vi "WPI_CameraSend Images to PC Loop_ONELOOP.vi"(6 "CameraDevRef Back":T1, 8 "error in (no error)":errorcluster, 9 "port":u16, 10 "Image Name":string, 11 "CameraDevRef Front":T1) -> ()   [LabVIEW 2015]
doc: "This VI is used to send images to the dashboard using the second enet port on the 8 slot controller. This is provided for compatibility, but is higher overhead than using the Camera MJPG approach.\n\nThis software is licensed. Open the labview\\readme\\WPI Robotics Library Open Source License.txt file for more information."
uses:
  <vilib>/Rock Robotics/WPI/Camera/WPI_CameraDevRef.ctl
  <vilib>/Rock Robotics/SystemInterfaces/NetworkCommunication/NetComm_UsageReport_ResourceType.ctl
  <vilib>/Rock Robotics/Network Tables/NT Read Boolean.vi
  Global Variables/Temp Variables.vi
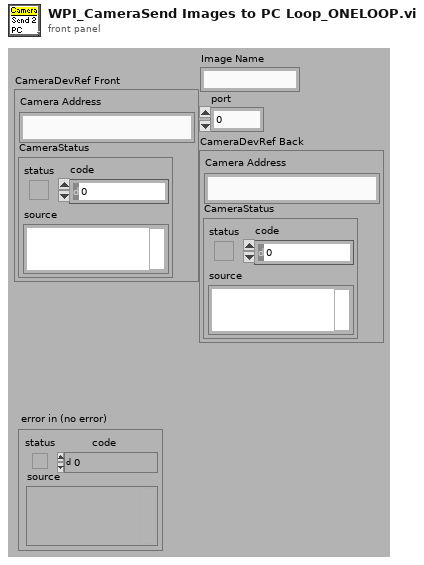
[diagram p1: front panel]
types:
  T1 = typedef "WPI_CameraDevRef.ctl" = cluster{"Camera Address":string, "CameraStatus":errorcluster}
  T2 = cluster{"fps":i32, "compression":i32, "compression 2":i32}
  T3 = typedef "NetComm_UsageReport_ResourceType.ctl" = enum8{"Controller", "Module", "Language", "CANPlugin", "Accelerometer", "ADXL345", "AnalogChannel", "AnalogTrigger", "AnalogTriggerOutput", "CANJaguar", "Compressor", "Counter", "Dashboard", "DigitalInput", "DigitalOutput", "DriverStationCIO", "DriverStationEIO", "DriverStationLCD", "Encoder", "GearTooth", "Gyro", "I2C", "Framework", "Jaguar", "Joystick", "Kinect", "KinectStick", "PIDController", "Preferences", "PWM", "Relay", "RobotDrive", "SerialPort", "Servo", "Solenoid", "SPI", "Task", "Ultrasonic", "Victor", "Button", "Command", "AxisCamera", "PCVideoServer", "SmartDashboard", "Talon", "HiTechnicColorSensor", "HiTechnicAccel", "HiTechnicCompass", "SRF08", "AnalogOutput", "Victor SP", "Talon SRX", "CAN Talon SRX", "ADXL362 Accel", "ADXRS450 Gyro", "Rev SPARK", "Mindsensors SD540", "Digital Filter"}
  T4 = enum16{"Update Mode", "Get Image", "Get Image Data"}
  T5 = typedef "Image Type" = u32
  T6 = typedef "IMAQ Image.ctl" = refnum<image>
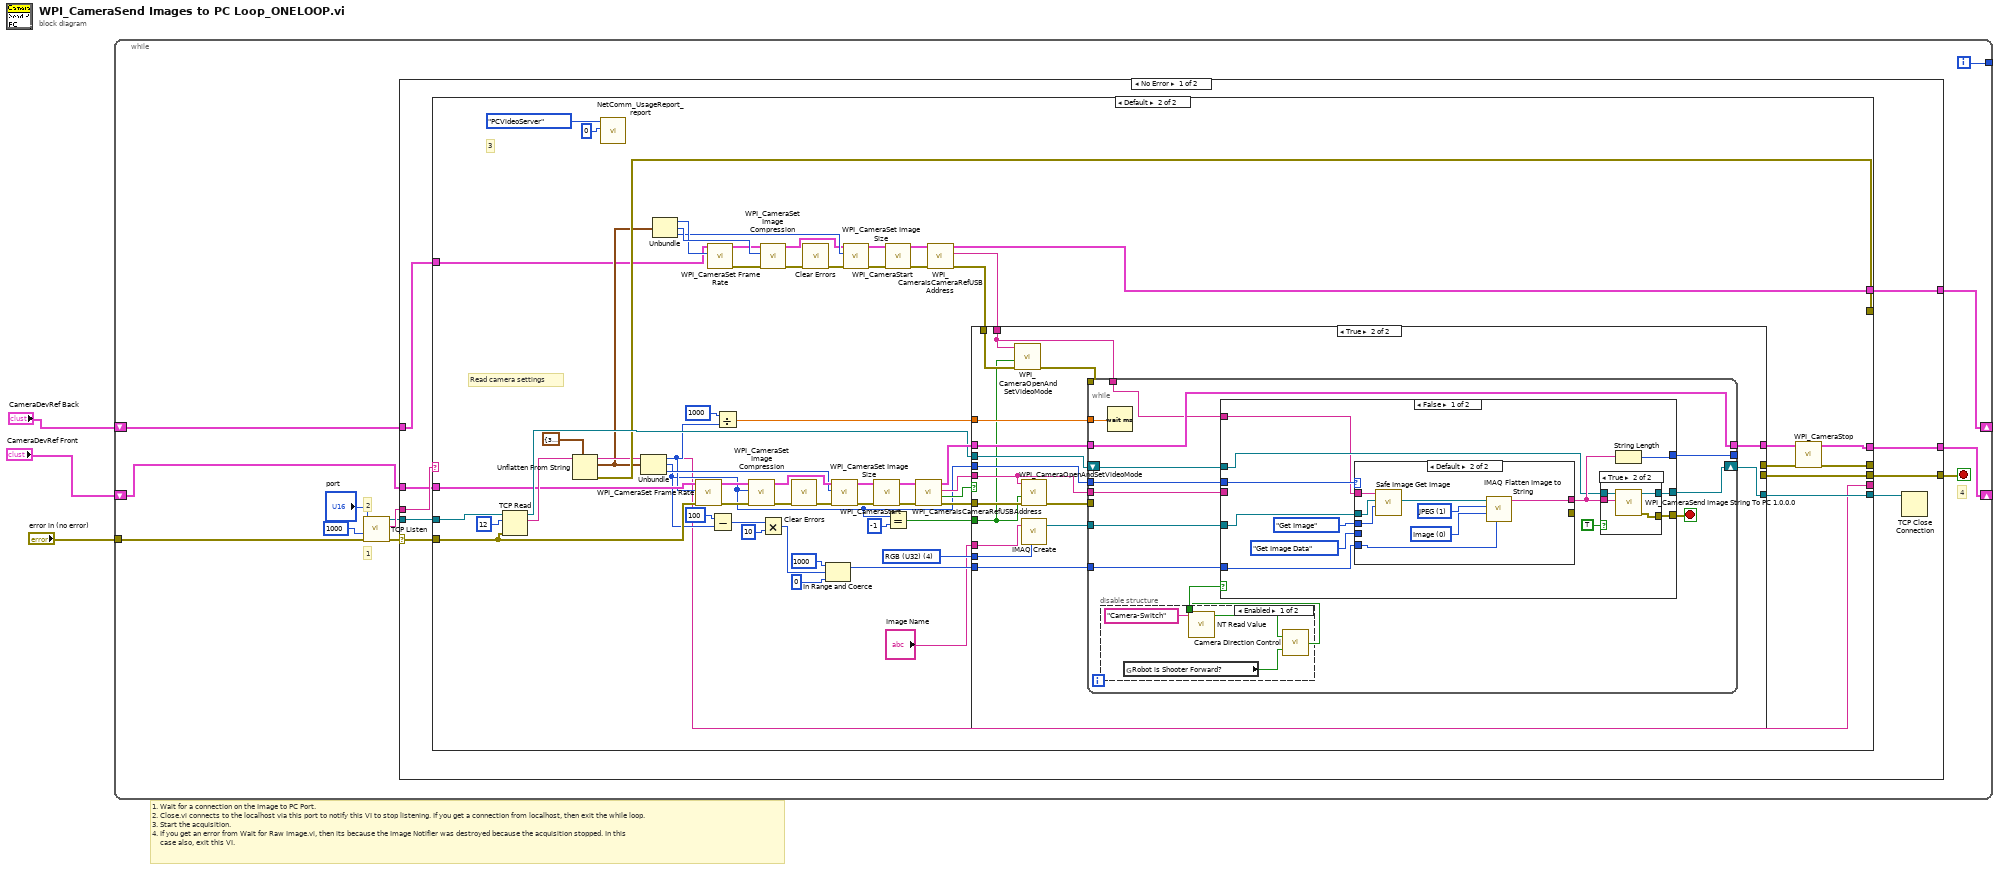
[diagram p0: block diagram]
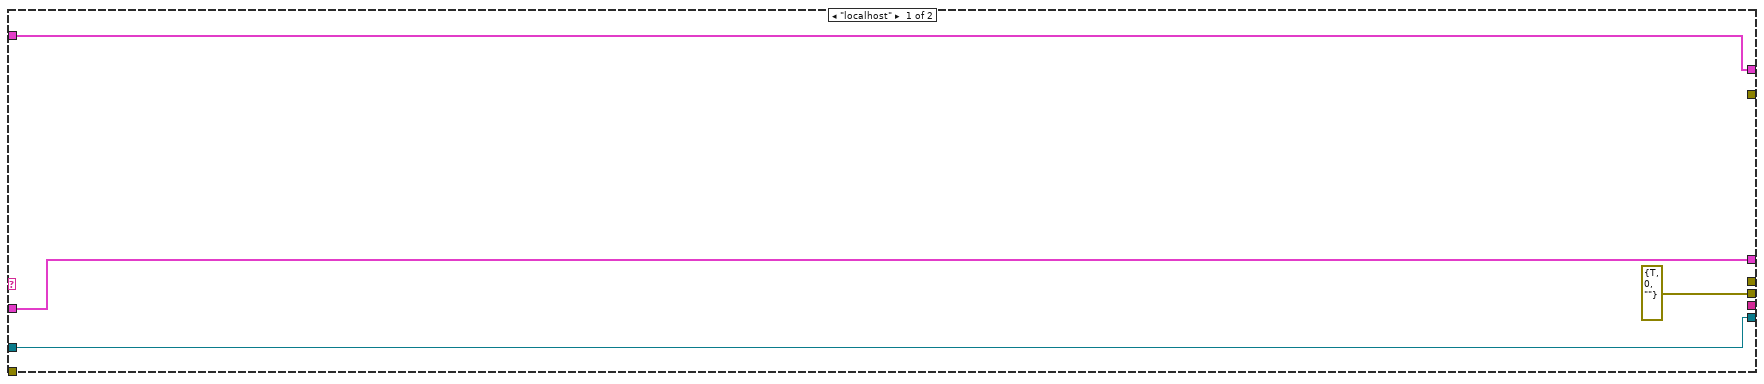
[diagram p2: hidden frame]
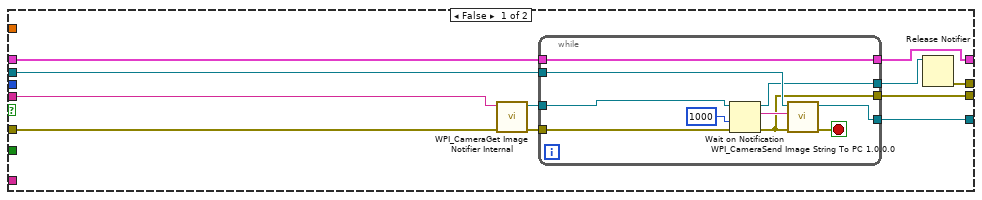
[diagram p3: hidden frame]
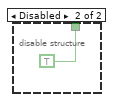
[diagram p4: hidden frame]
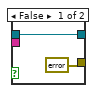
[diagram p5: hidden frame]
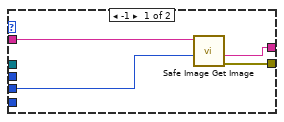
[diagram p6: hidden frame]
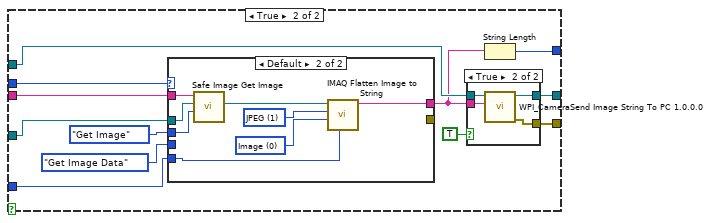
[diagram p7: hidden frame]
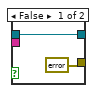
[diagram p8: hidden frame]
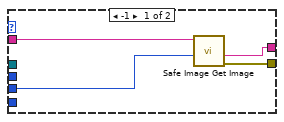
[diagram p9: hidden frame]
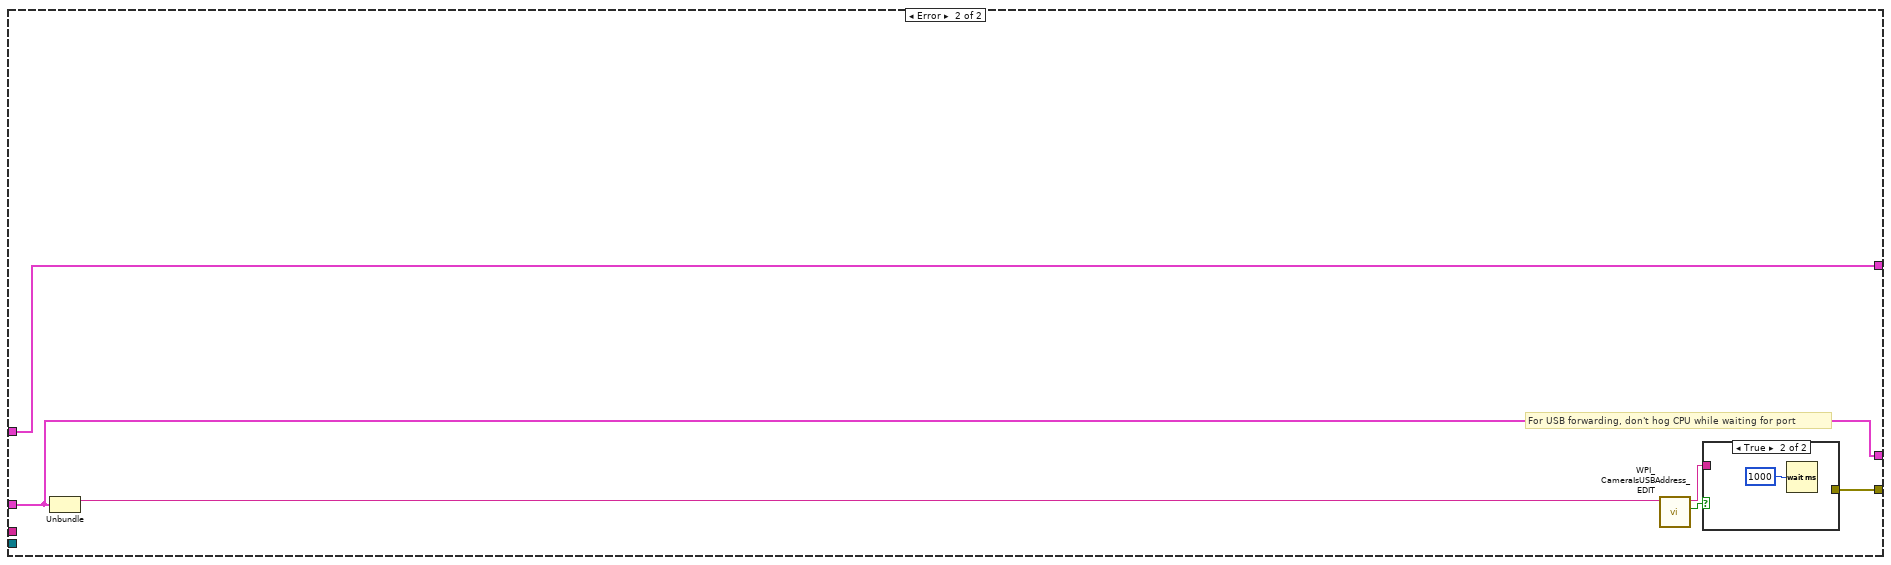
[diagram p10: hidden frame]
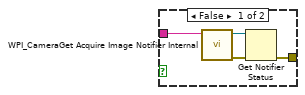
[diagram p11: hidden frame]
diagram:
  # "1. Wait for a connection on the Image to PC Port.\n2. Close.vi connects to the localhost via this port to notify this VI to stop listening. If you get a connection from localhost, then exit the while loop.\n3. Start the acquisition.\n4. If you get an error from Wait for Raw Image.vi, then its because the Image Notifier was destroyed because the acquisition stopped. In this\n    case also, exit this VI."
  n1 = while {
    tunnel: "error in (no error)" -> [w13]
    shift-right: [w15] -> _
    shift-left: "CameraDevRef Front" -> [w7]
    tunnel: [w8] -> _
    shift-right: [w4] -> _
    shift-left: "CameraDevRef Back" -> [w5]
    i -> [w8]
    stop <- w11 stop-if-true
    # "4"
    # "1"
    # "2"
    n2 = call <vilib>:"TCP Listen.vi"("error in (no error)"=w13, "timeout ms (wait forever: -1)"=u16 1000 ("port"), "port"="port") -> ("error out"=w10:errorcluster, "remote address"=w14:string, "connection ID"=w12:refnum<k5>)  [unwired: 1 in, 5 out]
    n3 = case shown="No Error" w10 {
      selector: w10 -> [w18 _]
      tunnel: [w24 w211] -> w15
      tunnel: w14 -> [w23 _]
      tunnel: w7 -> [w22 w211]
      tunnel: w12 -> [w21 _]
      tunnel: [w20 w212] -> w11
      tunnel: w5 -> [w17 w207]
      tunnel: [w16 w207] -> w4
      frame No Error {
        n4 = case shown="Default" w23 {
          tunnel: [w28 w89] -> w24
          tunnel: w22 -> [w28 w72]
          tunnel: w18 -> [_ w68]
          tunnel: w21 -> [w26 w76]
          tunnel: [errorcluster {"status"=TRUE, "code"=0, "source"=""} ("error out 2") w91] -> w20
          tunnel: [w26 w90] -> w19
          tunnel: [_ w88] -> _
          tunnel: [_ w48] -> _
          tunnel: [_ w47] -> _
          tunnel: w17 -> [w25 w32]
          tunnel: [w25 w29] -> w16
          frame "localhost" {
          }
          frame Default {
            w83 = T5 4 items=["Grayscale (U8)", "Grayscale (I16)", "Grayscale (SGL)", "Complex (CSG)", "RGB (U32)", "HSL (U32)", "RGB (U64)", "Grayscale (U16)"] ("Image Type")
            # "Read camera settings"
            # "3"
            n5 = TCP Read(connection ID=w76, bytes to read=12, error in (no error)=w68) -> (connection ID out=w75:refnum<k5>, data out=w73:string)  [unwired: 2 in, 1 out]
            n6 = Unflatten From String(type=T2 {"fps"=30, "compression"=32, "compression 2"=32} ("Camera Settings"), binary string=w73) -> (rest of the binary string=w47:string, value=w33:T2, error out=w48:errorcluster)  [unwired: 3 in]
            n7 = call <vilib>:"NetComm_UsageReport_report.vi"("Instance Number"=u8 0, "Resource Type"=NetComm_UsageReport_ResourceType."PCVideoServer") -> ()  [unwired: 10 in]
            n8 = Unbundle(w33) -> ("fps"=w63:i32, "compression"=w52:i32, "compression 2"=w65:i32)
            n9 = Unbundle(w33) -> ("fps"=w42:i32, "compression"=w43:i32, "compression 2"=w41:i32)
            n10 = call <vilib>:"WPI_CameraSet Frame Rate.vi"("error in (no error)"=w68, "Frame Rate (fps)"=w63, "CameraDevRef"=w72) -> ("error out"=w67:errorcluster, "CameraDevRef Out"=w71:T1)  [unwired: 7 in]
            n11 = call <vilib>:"WPI_CameraSet Frame Rate.vi"("Frame Rate (fps)"=w42, "CameraDevRef"=w32) -> ("error out"=w39:errorcluster, "CameraDevRef Out"=w36:T1)  [unwired: 8 in]
            n12 = Subtract(x=100, y=w52) -> (x-y=w57:i32)
            n13 = Divide(x=u16 1000 ("port"), y=w63) -> (x/y=w62:dbl)
            n14 = call <vilib>:"WPI_CameraSet Image Compression.vi"("error in (no error)"=w67, "Compression"=w52, "CameraDevRef"=w71) -> ("error out"=w50:errorcluster, "CameraDevRef Out"=w70:T1)  [unwired: 7 in]
            n15 = call <vilib>:"WPI_CameraSet Image Compression.vi"("error in (no error)"=w39, "Compression"=w43, "CameraDevRef"=w36) -> ("error out"=w44:errorcluster, "CameraDevRef Out"=w37:T1)  [unwired: 7 in]
            n16 = Multiply(x=w57, y=10) -> (x*y=w59:i32)
            n17 = call <vilib>:"Clear Errors.vi"("error in (no error)"=w50) -> ("error out"=w49:errorcluster)  [unwired: 5 in, 1 out]
            n18 = call <vilib>:"Clear Errors.vi"("error in (no error)"=w44) -> ("error out"=w45:errorcluster)  [unwired: 5 in, 1 out]
            n19 = In Range and Coerce(upper limit=1000, x=w59, lower limit=0) -> (coerced(x)=w55:i32)  [unwired: 1 out]
            n20 = call <vilib>:"WPI_CameraSet Image Size.vi"("error in (no error)"=w49, "Image Size"=w65, "CameraDevRef"=w70) -> ("error out"=w66:errorcluster, "CameraDevRef Out"=w69:T1)  [unwired: 7 in]
            n21 = call <vilib>:"WPI_CameraSet Image Size.vi"("error in (no error)"=w45, "Image Size"=w41, "CameraDevRef"=w37) -> ("error out"=w40:errorcluster, "CameraDevRef Out"=w38:T1)  [unwired: 7 in]
            n22 = call <vilib>:"WPI_CameraStart.vi"("error in (no error)"=w66, "CameraDevRef"=w69) -> ("error out"=w80:errorcluster, "CameraDevRef"=w78:T1)  [unwired: 8 out]
            n23 = call <vilib>:"WPI_CameraStart.vi"("error in (no error)"=w40, "CameraDevRef"=w38) -> ("error out"=w34:errorcluster, "CameraDevRef"=w35:T1)  [unwired: 8 out]
            n24 = Equal?(x=w52, y=-1) -> (x = y?=w51:bool)
            n25 = call <vilib>:"WPI_CameraIsCameraRefUSBAddress.vi"("error in (no error)"=w80, "CameraDevRef"=w78) -> ("error out"=w79:errorcluster, "USB?"=w81:bool, "Camera Address Out"=w82:string, "CameraDevRef out"=w77:T1)  [unwired: 6 in]
            n26 = call <vilib>:"WPI_CameraIsCameraRefUSBAddress.vi"("error in (no error)"=w34, "CameraDevRef"=w35) -> ("error out"=w30:errorcluster, "Camera Address Out"=w31:string, "CameraDevRef out"=w29:T1)  [unwired: 6 in, 1 out]
            n27 = case shown="True" w81 {
              tunnel: w75 -> [w102 w129]
              tunnel: [w101 _] -> w91
              tunnel: [w100 w128] -> w90
              tunnel: w79 -> [w99 w120]
              tunnel: w82 -> [w97 w119]
              tunnel: [w96 w124] -> w87
              tunnel: w77 -> [w95 w125]
              tunnel: [w93 _] -> w86
              tunnel: w83 -> [_ w126]
              tunnel: w55 -> [_ w123]
              tunnel: w62 -> [_ w122]
              tunnel: w52 -> [_ w121]
              tunnel: w51 -> [_ w115]
              tunnel: "Image Name" -> [_ w117]
              tunnel: w31 -> [_ w113]
              tunnel: w30 -> [_ w116]
              frame False {
                n28 = call <vilib>:"WPI_CameraGet Image Notifier Internal.vi"("error in (no error)"=w99, "Camera Address"=w97) -> ("error out"=w98:errorcluster, "Image Notifier"=w94:refnum<notifier>)  [unwired: 8 out]
                n29 = while {
                  tunnel: w98 -> [w108]
                  tunnel: w102 -> [w112]
                  tunnel: [w105] -> w101
                  tunnel: [w110] -> w100
                  tunnel: [w109] -> w96
                  tunnel: w95 -> [w109]
                  tunnel: w94 -> [w107]
                  tunnel: [w103] -> w92
                  stop <- w111 stop-if-true
                  n30 = Wait on Notification(notifier=w107, timeout in ms (-1)=1000 ("Timeout in ms (-1)"), error in (no error)=w108) -> (notifier out=w103:refnum<notifier>, notification=w106:string, error out=w105:errorcluster)  [unwired: 2 out]
                  n31 = call <vilib>:"WPI_CameraSend Image String To PC 1.0.0.0.vi"("error in (no error)"=w105, "String"=w106, "TCP Connection ID"=w112) -> ("error out"=w111:errorcluster, "TCP Connection ID out"=w110:refnum<k5>)  [unwired: 7 out]
                }
                n32 = Release Notifier(notifier=w92) -> (error out=w93:errorcluster)  [unwired: 1 in, 3 out]
              }
              frame True {
                n33 = call <vilib>:"WPI_CameraOpenAndSetVideoMode.vi"("error in (no error)"=w116, "USB JPEG"=w115, "Camera Address Out"=w113) -> ("error out"=w114:errorcluster)  [unwired: 8 in]
                n34 = call <vilib>:"WPI_CameraOpenAndSetVideoMode.vi"("error in (no error)"=w120, "USB JPEG"=w115, "Camera Address Out"=w119) -> ("error out"=w118:errorcluster)  [unwired: 8 in]
                n35 = call "IMAQ Create"("Image Name"=w117, "Image Type"=w126) -> ("New Image"=w127:T6)  [unwired: 3 in, 1 out]
                n36 = while {
                  tunnel: w119 -> [w140]
                  shift-right: [w141] -> w128
                  shift-left: w129 -> [w136]
                  tunnel: w127 -> [w139]
                  tunnel: [w132] -> w124
                  tunnel: w125 -> [w132]
                  tunnel: w123 -> [w138]
                  tunnel: w122 -> [w137]
                  tunnel: [w135] -> _
                  tunnel: w121 -> [w134]
                  tunnel: w118 -> [_]
                  tunnel: w114 -> [_]
                  tunnel: w113 -> [w131]
                  stop <- w133 stop-if-true
                  n37 = disable-structure shown="Enabled" {
                    disable-tunnel: [w142 TRUE] -> w130
                    frame Enabled {
                      n38 = global read "Temp Variables.vi" "Robot is Shooter Forward?"() -> (w144:bool)
                      n39 = call-poly <vilib>:"NT Read Value.vi"("Name"="Camera-Switch") -> ("Boolean"=w143:bool)  [unwired: 9 in, 1 out]
                      n40 = call "Camera Direction Control.vi"("Current Driving Direction (True = Shooter Forward)"=w144, "Camera Switch"=w143) -> ("Camera Direction (True = Shooter Camera)"=w142:bool)
                    }
                    frame Disabled {
                    }
                  }
                  n41 = Wait (ms)(milliseconds to wait=w137) -> ()  [unwired: 1 out]
                  n42 = case shown="False" w130 {
                    tunnel: [w149 w188] -> w141
                    tunnel: w140 -> [_ w187]
                    tunnel: w139 -> [w153 w186]
                    tunnel: w138 -> [w154 w185]
                    tunnel: w136 -> [w152 w184]
                    tunnel: [w150 w183] -> w135
                    tunnel: w134 -> [w151 w182]
                    tunnel: [w147 w179] -> w133
                    tunnel: w131 -> [w148 _]
                    frame False {
                      n43 = case shown="Default" w151 {
                        tunnel: [w167 w176] -> w157
                        tunnel: w148 -> [w168 w172]
                        tunnel: w153 -> [_ w171]
                        tunnel: w154 -> [_ w173]
                        tunnel: [w166 _] -> _
                        tunnel: T4."Get Image Data" ("Operation") -> [w165 _]
                        tunnel: T4."Get Image" ("Operation") -> [_ w169]
                        frame -1 {
                          n44 = call <vilib>:"Safe Image Get Image.vi"("Operation"=w165, "Session In"=w168) -> ("error out"=w166:errorcluster, "Image Data String"=w167:string)  [unwired: 6 in, 2 out]
                        }
                        frame Default {
                          w174 = 0 items=["Image", "Image and Vision Info", "Reference to Image"] ("Type of Flatten (Image and Vision Info)")
                          w175 = 1 items=["None", "JPEG", "PACKED BINARY"] ("Compression (None)")
                          n45 = call <vilib>:"Safe Image Get Image.vi"("Operation"=w169, "Image In"=w171, "Session In"=w172) -> ("Image Out"=w170:T6)  [unwired: 5 in, 3 out]
                          n46 = call "IMAQ Flatten Image to String"("Quality (750)"=w173, "Type of Flatten (Image and Vision Info)"=w174, "Compression (None)"=w175, "Image"=w170) -> ("Data String"=w176:string)  [unwired: 6 in, 1 out]
                        }
                      }
                      n47 = case shown="True" TRUE {
                        tunnel: [w160 w164] -> w149
                        tunnel: w152 -> [w160 w163]
                        tunnel: [errorcluster {"status"=FALSE, "code"=0, "source"=""} ("error out") w162] -> w147
                        tunnel: w157 -> [_ w161]
                        frame False {
                        }
                        frame True {
                          n48 = call <vilib>:"WPI_CameraSend Image String To PC 1.0.0.0.vi"("String"=w161, "TCP Connection ID"=w163) -> ("error out"=w162:errorcluster, "TCP Connection ID out"=w164:refnum<k5>)  [unwired: 1 in, 7 out]
                        }
                      }
                      n49 = String Length(string=w157) -> (length=w150:i32)
                    }
                    frame True {
                      n50 = case shown="Default" w182 {
                        tunnel: [w197 w206] -> w178
                        tunnel: w187 -> [w198 w202]
                        tunnel: w186 -> [_ w201]
                        tunnel: w185 -> [_ w203]
                        tunnel: [w196 _] -> _
                        tunnel: T4."Get Image Data" ("Operation") -> [w195 _]
                        tunnel: T4."Get Image" ("Operation") -> [_ w199]
                        frame -1 {
                          n51 = call <vilib>:"Safe Image Get Image.vi"("Operation"=w195, "Session In"=w198) -> ("error out"=w196:errorcluster, "Image Data String"=w197:string)  [unwired: 6 in, 2 out]
                        }
                        frame Default {
                          w204 = 0 items=["Image", "Image and Vision Info", "Reference to Image"] ("Type of Flatten (Image and Vision Info)")
                          w205 = 1 items=["None", "JPEG", "PACKED BINARY"] ("Compression (None)")
                          n52 = call <vilib>:"Safe Image Get Image.vi"("Operation"=w199, "Image In"=w201, "Session In"=w202) -> ("Image Out"=w200:T6)  [unwired: 5 in, 3 out]
                          n53 = call "IMAQ Flatten Image to String"("Quality (750)"=w203, "Type of Flatten (Image and Vision Info)"=w204, "Compression (None)"=w205, "Image"=w200) -> ("Data String"=w206:string)  [unwired: 6 in, 1 out]
                        }
                      }
                      n54 = case shown="True" TRUE {
                        tunnel: [w190 w194] -> w188
                        tunnel: w184 -> [w190 w193]
                        tunnel: [errorcluster {"status"=FALSE, "code"=0, "source"=""} ("error out") w192] -> w179
                        tunnel: w178 -> [_ w191]
                        frame False {
                        }
                        frame True {
                          n55 = call <vilib>:"WPI_CameraSend Image String To PC 1.0.0.0.vi"("String"=w191, "TCP Connection ID"=w193) -> ("error out"=w192:errorcluster, "TCP Connection ID out"=w194:refnum<k5>)  [unwired: 1 in, 7 out]
                        }
                      }
                      n56 = String Length(string=w178) -> (length=w183:i32)
                    }
                  }
                }
              }
            }
            n57 = call <vilib>:"WPI_CameraStop.vi"("error in (no error)"=w86, "CameraDevRef"=w87) -> ("error out"=w88:errorcluster, "CameraDevRef"=w89:T1)  [unwired: 8 out]
          }
        }
        n58 = TCP Close Connection(connection ID=w19) -> ()  [unwired: 1 in, 3 out]
      }
      frame Error {
        # "For USB forwarding, don't hog CPU while waiting for port"
        n59 = Unbundle(w211) -> ("Camera Address"=w210:string)  [unwired: 1 out]
        n60 = call "WPI_CameraIsUSBAddress_EDIT.vi"("Camera Address In"=w210) -> ("USB?"=w208:bool, "Camera Address Out"=w209:string)  [unwired: 8 in, 1 out]
        n61 = case shown="True" w208 {
          tunnel: [w216 _] -> w212
          tunnel: w209 -> [w213 _]
          frame False {
            n62 = call <vilib>:"WPI_CameraGet Acquire Image Notifier Internal.vi"("Camera Address"=w213) -> ("error out"=w214:errorcluster, "Acquire Image Notifier"=w215:refnum<notifier>)  [unwired: 1 in, 8 out]
            n63 = Get Notifier Status(notifier=w215, error in (no error)=w214) -> (error out=w216:errorcluster)  [unwired: 4 out]
          }
          frame True {
            n64 = Wait (ms)(milliseconds to wait=u32 1000) -> ()  [unwired: 1 out]
          }
        }
      }
    }
  }
